vi "Conversion main.vi"(8 "error in (no error)":errorcluster, 11 "DAQMH121119OrcaFlash in":refnum<class "DAQOrcaFlash.lvclass">) -> (0 "error out":errorcluster, 3 "DAQMH121119OrcaFlash out":refnum<class "DAQOrcaFlash.lvclass">)   [LabVIEW 2012, in "DAQOrcaFlash.lvclass"]
uses:
  DAQOrcaFlash.lvclass
  conversion_work_queue.ctl
  class variable.vi
panel:
  in  "start":bool
  out "paths":path[](array[path])
  out "filename":string
  out "progress bar":sgl(slide) scale=0.0..1.0 scale format="%3.0f"
  in  "stop":bool
  in  "path out":path
  in  "path in":path
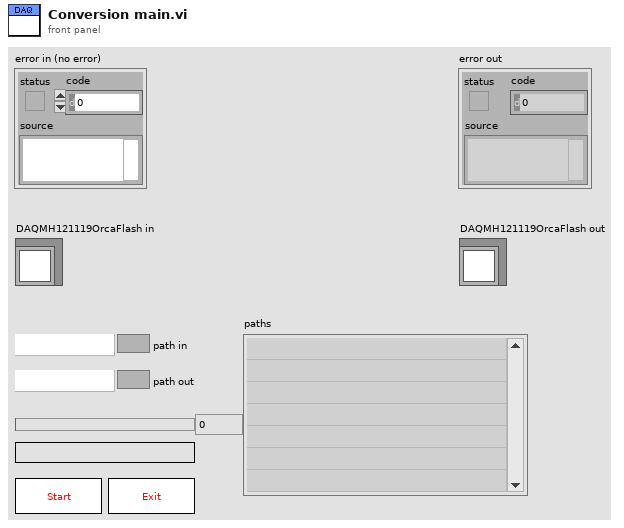
[diagram p1: front panel]
types:
  T1 = typedef "DAQOrcaFlash.lvclass/conversion_work_queue.ctl" = cluster{"origin":path, "destination":path}
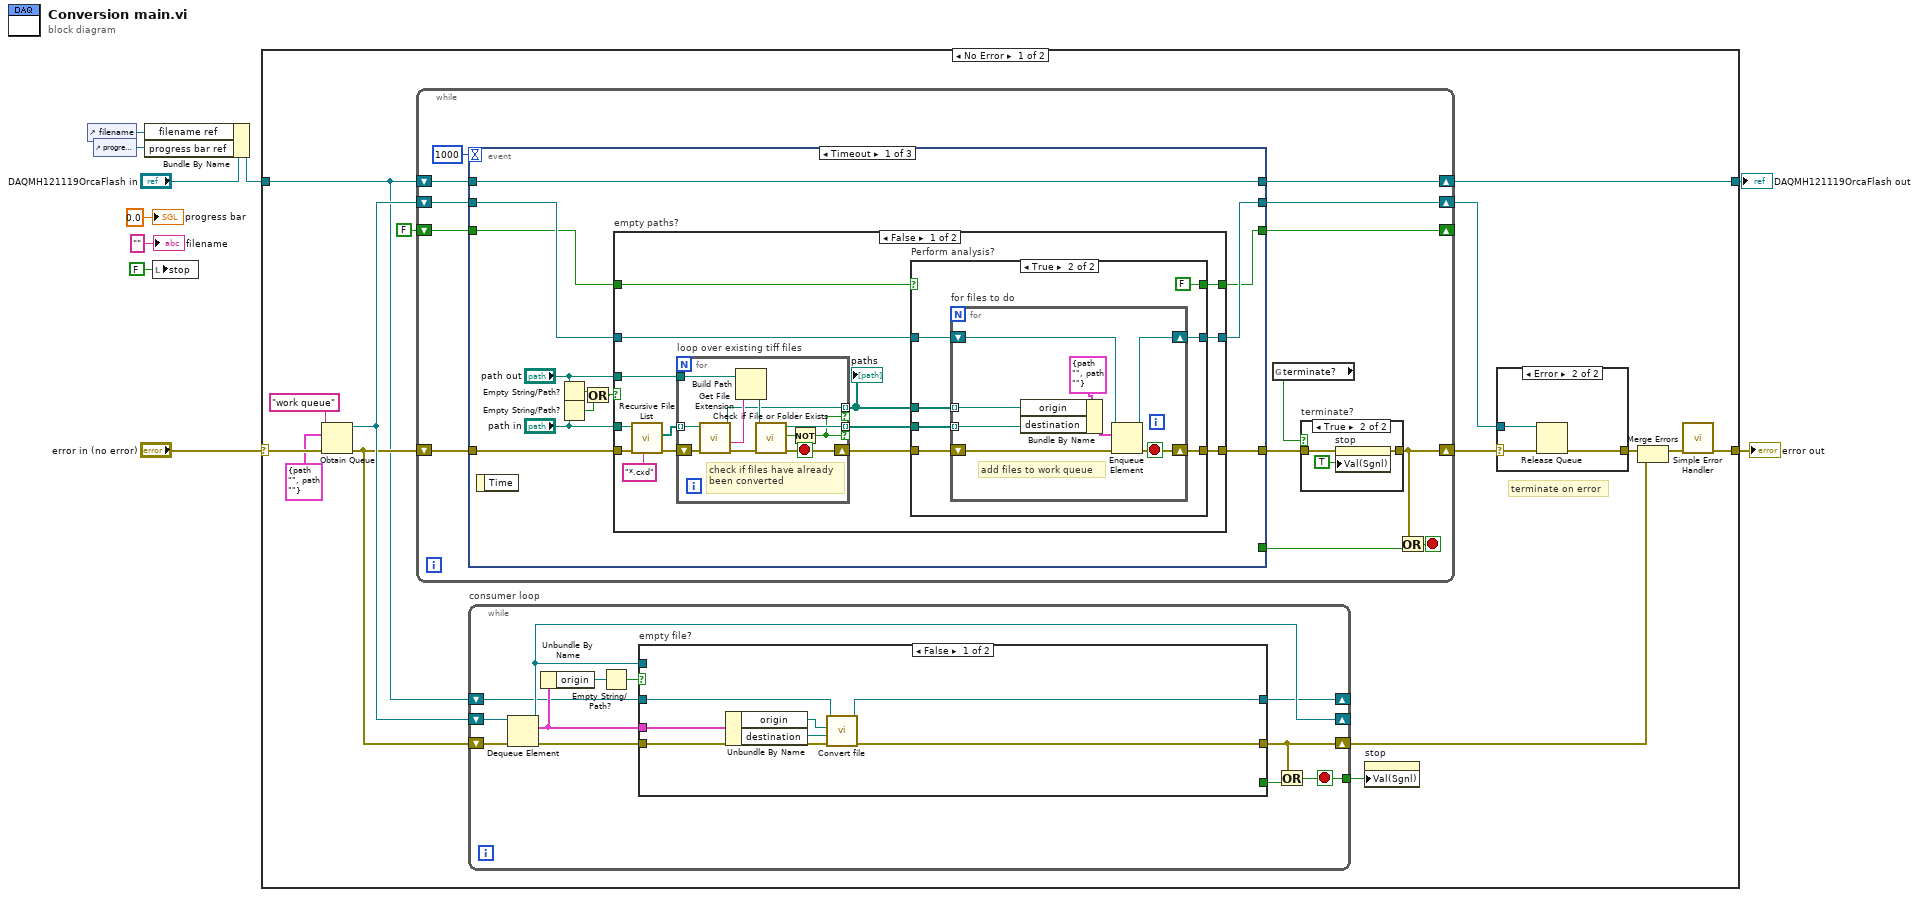
[diagram p0: block diagram]
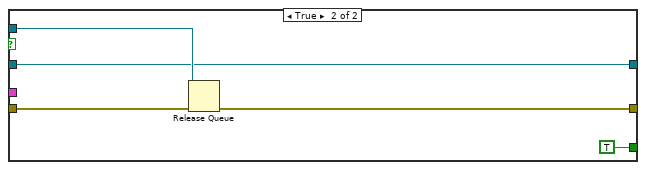
[diagram p3: hidden frame]
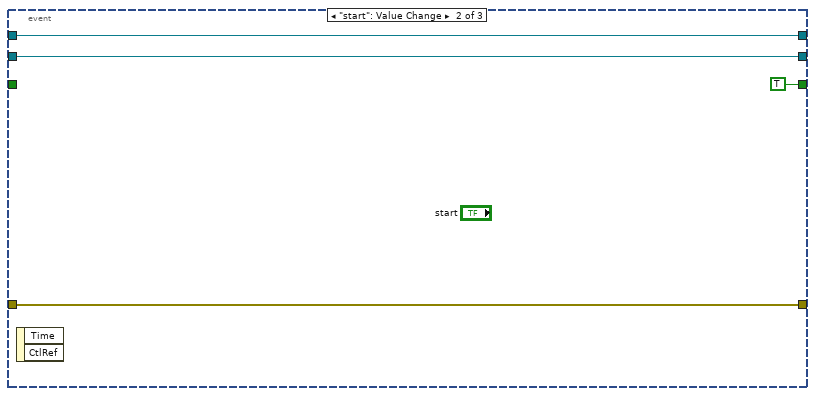
[diagram p7: hidden frame]
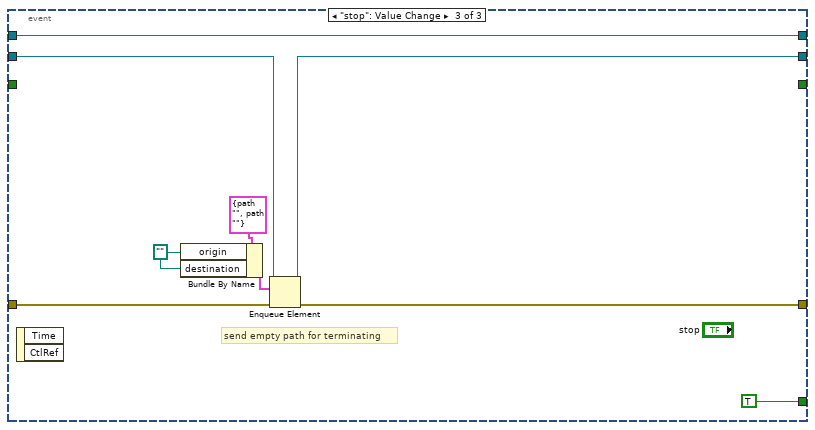
[diagram p8: hidden frame]
diagram:
  n1 = control-ref of="filename"() -> (w5:refnum<vi>)
  n2 = control-ref of="progress bar"() -> (w8:refnum<vi>)
  n3 = Bundle By Name(cluster="DAQMH121119OrcaFlash in", "filename ref"=w5, "progress bar ref"=w8) -> (w6:refnum<class "DAQOrcaFlash.lvclass">)
  n4 = local write "stop"(FALSE ("stop")) -> ()
  n5 = case shown="No Error" "error in (no error)" {
    selector: "error in (no error)" -> [w24 w142]
    tunnel: [w14 w142] -> w1
    tunnel: [w25 w141] -> w9
    tunnel: w6 -> [w19 w141]
    frame No Error {
      # "terminate on error"
      n6 = Obtain Queue(name (unnamed)="work queue", element data type=T1 {"origin"=path "", "destination"=path ""}, error in (no error)=w24) -> (queue out=w21:refnum<queue>, error out=w20:errorcluster)  [unwired: 2 in, 1 out]
      n7 = while {
        shift-right: [w55] -> w13
        shift-left: w20 -> [w66]
        shift-right: [w65] -> w25
        shift-left: w19 -> [w64]
        shift-right: [w61] -> w11
        shift-left: w21 -> [w62]
        shift-right: [w58] -> _
        shift-left: FALSE -> [w57]
        stop <- w59 stop-if-true
        n8 = event shown="[0] Timeout" {
          selector: _ -> [_ _ _]
          dyn-events: _ -> [_ _ _]
          timeout: 1000 -> [_ _ _]
          tunnel: [w80 w129 w137] -> w54
          tunnel: w66 -> [w81 w129 w138]
          tunnel: [w82 w131 w140] -> w65
          tunnel: w64 -> [w82 w131 w140]
          tunnel: w62 -> [w78 w130 w136]
          tunnel: [w79 w130 w135] -> w61
          tunnel: [_ _ TRUE] -> w60
          tunnel: [w76 TRUE _] -> w58
          tunnel: w57 -> [w77 _ _]
          event Timeout {
            n9 = event-data() -> ()  [unwired: 1 in, 1 out]
            n10 = Empty String/Path?(string/path="path out") -> (empty?=w73:bool)
            n11 = Empty String/Path?(string/path="path in") -> (empty?=w72:bool)
            n12 = Or(x=w73, y=w72) -> (x .or. y?=w71:bool)
            n13 = case "empty paths?" shown="False" w71 {
              tunnel: w81 -> [w96 w127]
              tunnel: [w91 w127] -> w80
              tunnel: [w90 w126] -> w79
              tunnel: w78 -> [w89 w126]
              tunnel: w77 -> [w86 w125]
              tunnel: [w85 w125] -> w76
              tunnel: "path in" -> [w84 _]
              tunnel: "path out" -> [w83 _]
              frame False {
                n14 = call <vilib>:"Recursive File List.vi"("pattern"="*.cxd", "error in (no error)"=w96, "Folder Path"=w84) -> ("error out"=w94:errorcluster, "All Files in Dir"=w88:path[])  [unwired: 4 in, 3 out]
                n15 = for "loop over existing tiff files" {
                  shift-right: [w116] -> w92
                  shift-left: w94 -> [w124]
                  tunnel: w88 -> [w123] mode=indexing
                  tunnel: w83 -> [w122]
                  tunnel: [w118] -> w93 mode=indexing if=w114
                  tunnel: [w115] -> w87 mode=indexing if=w114
                  stop <- w116 stop-if-true
                  # "check if files have already\nbeen converted"
                  n16 = call <vilib>:"Get File Extension.vi"("error in (no error)"=w124, "file"=w123) -> ("error out"=w120:errorcluster, "filename without extension"=w121:string, "dup file"=w115:path)  [unwired: 6 in, 1 out]
                  n17 = Build Path(base path=w122, name or relative path=w121) -> (appended path=w119:path)
                  n18 = call <vilib>:"Check if File or Folder Exists.vi"("error in (no error)"=w120, "path"=w119) -> ("error out"=w116:errorcluster, "file or folder exists?"=w117:bool, "dup path"=w118:path)  [unwired: 7 in]
                  n19 = Not(x=w117) -> (.not. x?=w114:bool)
                }
                "paths" <- w87
                n20 = case "Perform analysis?" shown="True" w86 {
                  tunnel: w93 -> [_ w105]
                  tunnel: w92 -> [w97 w104]
                  tunnel: [w97 w103] -> w91
                  tunnel: w87 -> [_ w102]
                  tunnel: [w98 w101] -> w90
                  tunnel: w89 -> [w98 w100]
                  tunnel: [_ FALSE] -> w85
                  frame False {
                  }
                  frame True {
                    n21 = for "for files to do" {
                      tunnel: w105 -> [w106] mode=indexing
                      shift-right: [w113] -> w103
                      shift-left: w104 -> [w107]
                      tunnel: w102 -> [w109] mode=indexing
                      shift-right: [w112] -> w101
                      shift-left: w100 -> [w111]
                      stop <- w113 stop-if-true
                      # "add files to work queue"
                      n22 = Bundle By Name(cluster=T1 {"origin"=path "", "destination"=path ""}, "origin"=w109, "destination"=w106) -> (w108:T1)
                      n23 = Enqueue Element(queue=w111, element=w108, error in (no error)=w107) -> (queue out=w112:refnum<queue>, error out=w113:errorcluster)  [unwired: 1 in, 1 out]
                    }
                  }
                }
              }
              frame True {
              }
            }
          }
          event "start": Value Change {
            n24 = event-data() -> ()  [unwired: 1 in, 2 out]
          }
          event "stop": Value Change {
            w133 = path ""
            # "send empty path for terminating"
            n25 = event-data() -> ()  [unwired: 1 in, 2 out]
            n26 = Bundle By Name(cluster=T1 {"origin"=path "", "destination"=path ""}, "origin"=w133, "destination"=w133) -> (w132:T1)
            n27 = Enqueue Element(queue=w136, element=w132, error in (no error)=w138) -> (queue out=w135:refnum<queue>, error out=w137:errorcluster)  [unwired: 1 in, 1 out]
          }
        }
        n28 = global read "class variable.vi" "terminate?"() -> (w56:bool)
        n29 = case "terminate?" shown="True" w56 {
          tunnel: [w67 w69] -> w55
          tunnel: w54 -> [w67 w68]
          frame False {
          }
          frame True {
            n30 = property on="stop" class="Bool (strict)"(error in=w68, "Val(Sgnl)"=TRUE ("Value (Signaling)")) -> (error out=w69:errorcluster)  [unwired: 1 in, 1 out]
          }
        }
        n31 = Or(x=w55, y=w60) -> (x .or. y?=w59:bool)
      }
      n32 = while "consumer loop" {
        shift-right: [w37] -> _
        shift-left: w21 -> [w41]
        shift-right: [w34] -> w17
        shift-left: w20 -> [w40]
        shift-right: [w31] -> _
        shift-left: w19 -> [w32]
        tunnel: [w30] -> w16
        stop <- w30 stop-if-true
        n33 = Dequeue Element(queue=w41, error in (no error)=w40) -> (queue out=w37:refnum<queue>, element=w35:T1, error out=w36:errorcluster)  [unwired: 1 in, 1 out]
        n34 = Unbundle By Name(w35) -> ("origin"=w39:path)
        n35 = Empty String/Path?(string/path=w39) -> (empty?=w38:bool)
        n36 = case "empty file?" shown="False" w38 {
          tunnel: w37 -> [_ w53]
          tunnel: w36 -> [w47 w52]
          tunnel: [w46 w51] -> w34
          tunnel: w35 -> [w48 _]
          tunnel: [_ TRUE] -> w33
          tunnel: w32 -> [w43 w49]
          tunnel: [w42 w49] -> w31
          frame False {
            n37 = Unbundle By Name(w48) -> ("origin"=w44:path, "destination"=w45:path)
            n38 = call "Convert file.vi"("error in (no error)"=w47, "file out"=w45, "file in"=w44, "DAQMH121119OrcaFlash in"=w43) -> ("error out"=w46:errorcluster, "DAQMH121119OrcaFlash out"=w42:refnum<class "DAQOrcaFlash.lvclass">)  [unwired: 6 in]
          }
          frame True {
            n39 = Release Queue(queue=w53, error in (no error)=w52) -> (error out=w51:errorcluster)  [unwired: 1 in, 2 out]
          }
        }
        n40 = Or(x=w34, y=w33) -> (x .or. y?=w30:bool)
      }
      n41 = property on="stop" class="Bool (strict)"("Val(Sgnl)"=w16) -> ()  [unwired: 2 in, 2 out]
      n42 = case shown="Error" w13 {
        selector: w13 -> [w26 w29]
        tunnel: [w26 w28] -> w12
        tunnel: w11 -> [_ w27]
        frame No Error {
        }
        frame Error {
          n43 = Release Queue(queue=w27, error in (no error)=w29) -> (error out=w28:errorcluster)  [unwired: 1 in, 2 out]
        }
      }
      n44 = Merge Errors(w12, w17) -> (w15:errorcluster)
      n45 = call <vilib>:"Simple Error Handler.vi"("error in (no error)"=w15) -> ("error out"=w14:errorcluster)  [unwired: 4 in, 4 out]
    }
    frame Error {
    }
  }
  "error out" <- w1
  "DAQMH121119OrcaFlash out" <- w9
  "progress bar" <- sgl 0.0 ("progress bar")
  "filename" <- "" ("filename")
